vi "SPI Init.vi"(9 "pConfig":T1, 10 "SPIIndex":i32, 11 "DevIndex":i32) -> (3 "function return":i32)   [LabVIEW 2010, in "usb2spi.lvlib"]
doc: "int WINAPI SPI_Init(int DevIndex,int SPIIndex, PSPI_CONFIG pConfig);"
uses:
  usb2spi.lvlib
  USB2XXX.dll
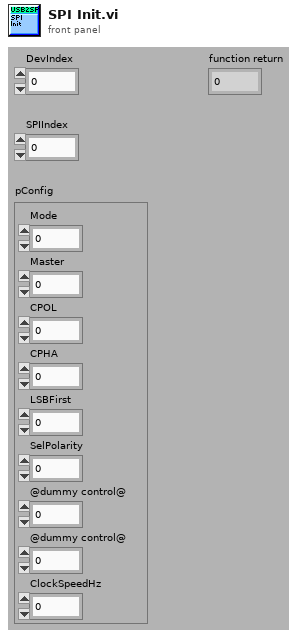
[diagram p1: front panel]
types:
  T1 = cluster{"Mode":i8, "Master":i8, "CPOL":i8, "CPHA":i8, "LSBFirst":i8, "SelPolarity":i8, "@dummy control@":i8, "@dummy control@":i8, "ClockSpeedHz":u32}
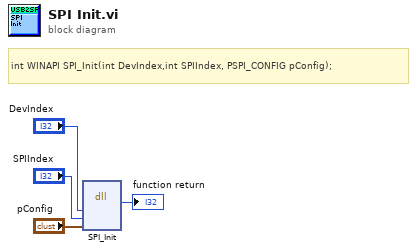
[diagram p0: block diagram]
diagram:
  # "int WINAPI SPI_Init(int DevIndex,int SPIIndex, PSPI_CONFIG pConfig);"
  n1 = dll-call lib="G:/OtherWork/USB2XXX_Example/trunk/Labview/PublicFiles/usb2spi/USB2XXX.*" fn="SPI_Init"("DevIndex"="DevIndex", "SPIIndex"="SPIIndex", "pConfig"="pConfig") -> (→"function return":i32)  [unwired: 6 in, 2 out]
